vi "sub vi - AI USB4704 (3)  Close Task v2.vi"   [LabVIEW 2017]
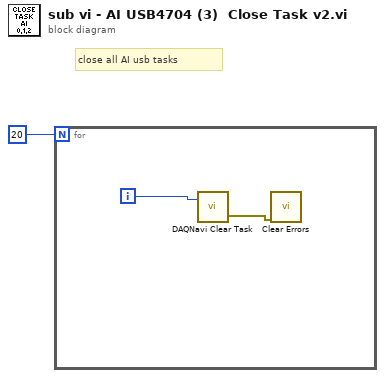
[diagram p0: block diagram]
diagram:
  # "close all AI usb tasks"
  n1 = for {
    N: 20 -> [_]
    i -> [w3]
    n2 = call <userlib>:"DAQNavi Clear Task.vi"("task in"=w3) -> ("error out"=w2:errorcluster)  [unwired: 1 in, 1 out]
    n3 = call <vilib>:"Clear Errors.vi"("error in (no error)"=w2) -> ()  [unwired: 5 in, 2 out]
  }
